vi "WPI_CANTalonSRX_Send.vi"(11 "Device ID (0)":u8) -> (3 "Device ID Out":u8)   [LabVIEW 2016]
uses:
  <vilib>/Rock Robotics/WPI/ThirdParty/CanMotor/TalonSRX/WPI_CANTalonSRX_GlobalOps.ctl
  <vilib>/Rock Robotics/WPI/ThirdParty/CanMotor/TalonSRX/WPI_CANTalonSRX_GlobalStatus.ctl
  <vilib>/Rock Robotics/WPI/ThirdParty/CanMotor/TalonSRX/WPI_CANTalonSRX_APIControlMode.ctl
  <vilib>/Rock Robotics/WPI/ThirdParty/CanMotor/TalonSRX/WPI_CANTalonSRX_ControlMode.ctl
  <vilib>/Rock Robotics/WPI/ThirdParty/CanMotor/TalonSRX/WPI_CANTalonSRX_MessageIDs.ctl
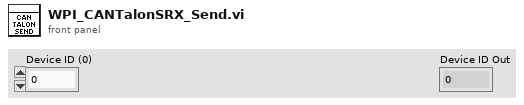
[diagram p1: front panel]
types:
  T1 = typedef "WPI_CANTalonSRX_APIControlMode.ctl" = enum8{"Percent VBus", "Speed", "Position", "Slave", "Unchanged / Invalid", "Voltage Compensation", "Current", "Motion Profile", "Motion Magic"}
  T2 = typedef "WPI_CANTalonSRX_GlobalOps.ctl" = enum16{"Read For Send", "Write After Receive General", "Write After Receive Feedback", "Write After Receive Encoder", "Write After Receive Ain", "Write Error", "Get All", "Set Output", "Set Mode", "Set Master ID", "Set Brake Mode", "Set Reverse Feedback Sensor", "Set Reverse Closed Loop Output", "Set Override Limits", "Set Forward Limit Enabled", "Set Reverse Limit Enabled", "Set Feedback Select", "Set Profile Select", "Set Throttle Ramp Rate", "Disable", "Set Enc Codes Per Rev", "Set Num Pot Turns", "Set Control Frame Rate", "Enable Legacy Control", "Write After Receive Pulse Width", "Set Enable Frame Rate", "Write After Receive Motion Profile", "Set Motion Profile Flow Control", "Set Motion Profile Control Frame Rate", "Set Current Limit Enable"}
  T3 = typedef "WPI_CANTalonSRX_GlobalStatus.ctl" = cluster{"Applied Throttle":dbl, "Module Enabled":bool, "CAN Error":errorcluster, "Closed Loop Error":dbl, "Forward Limit Switch Closed":bool, "Reverse Limit Switch Closed":bool, "Sensor Position":dbl, "Sensor Velocity":dbl, "Current":dbl, "Sticky Fault - Over Temp":bool, "Sticky Fault - Under Voltage":bool, "Sticky Fault - Forward Limit":bool, "Sticky Fault - Reverse Limit":bool, "Sticky Fault - Forward Soft Limit":bool, "Sticky Fault - Reverse Soft Limit":bool, "Brake is Enabled":bool, "Encoder Position":dbl, "Encoder Velocity":dbl, "Encoder Index Count":dbl, "Encoder A Pin State":bool, "Encoder B Pin State":bool, "Encoder Index Pin State":bool, "Analog In":dbl, "Analog In Velocity":dbl, "Temperature (C)":dbl, "Battery Voltage":dbl, "Control 5 Is Supported":bool, "Current Profile Slot Select":dbl, "Pos Div 8":bool, "Vel Div 4":bool, "Pulse Width Position":i32, "Pulse Width Velocity":i32, "Pulse Width Rise To Rise (us)":i32, "Pulse Width Rise To Fall (us)":i32, "Mot Prof Active Is Under Run":bool, "Mot Prof Active Has Under Run":bool, "Mot Prof Active Is Last":bool, "Mot Prof Active Velocity Only":bool, "Mot Prof Active Is Valid":bool, "Mot Prof Buffer Is Full":bool, "Mot Prof Active Profile Slot Select":i32, "Mot Prof NextID":i32, "Mot Prof Count":i32, "Mot Prof Active Velocity":dbl, "Mot Prof Active Position":dbl, "Mot Prof Output Enable":i32}
  T4 = typedef "WPI_CANTalonSRX_GlobalControl.ctl" = cluster{"Output":dbl, "Control Mode":T1, "Brake-Mode Override":T5, "Reverse Feedback Sensor":bool, "Reverse Closed-Loop Output":bool, "Override Limits":bool, "Forward Limit Enabled":bool, "Reverse Limit Enabled":bool, "Feedback Select":T6, "Profile Select":u8, "Master To Follow":u8, "Throttle Ramp Rate":u8, "Disabled":bool, "Encoder Codes Per Rev":u32, "Num Pot Turns":u32, "Control Frame Rate Ms":u8, "Use Control5 If Supported":bool, "Enable Frame Rate Ms":u8, "Motion Profile Flow Control":u8, "Motion Profile Control Frame Rate":u8, "Talon SRX Motion Profile Trajectory Point":T7, "Current Limit Enabled":bool}
  T5 = typedef "WPI_CANTalonSRX_BrakeOverride.ctl" = enum8{"No Override", "Override to Coast", "Override to Brake"}
  T6 = typedef "WPI_CANTalonSRX_FeedbackSelect.ctl" = u8
  T7 = typedef "WPI_CANTalonSRX_MotionProfileTrajectoryPt.ctl" = cluster{"Duration Ms":u8, "Velocity":dbl, "Position":dbl, "Profile Slot Select":u8, "Is Last":bool, "Velocity Only":bool, "Zero Position":bool, "Compress Code":u8, "Same Velocity":i32, "Delta Position":i32, "Count":u8}
  T8 = typedef "WPI_CANTalonSRX_ControlMode.ctl" = enum16{"Throttle (Duty-Cycle)", "Position Closed-Loop", "Velocity Closed-Loop", "Current Closed-Loop", "Voltage Compensation", "Slave Follower", "Motion Profile", "Motion Magic"}
  T9 = typedef "WPI_CANTalonSRX_MessageIDs.ctl" = u32
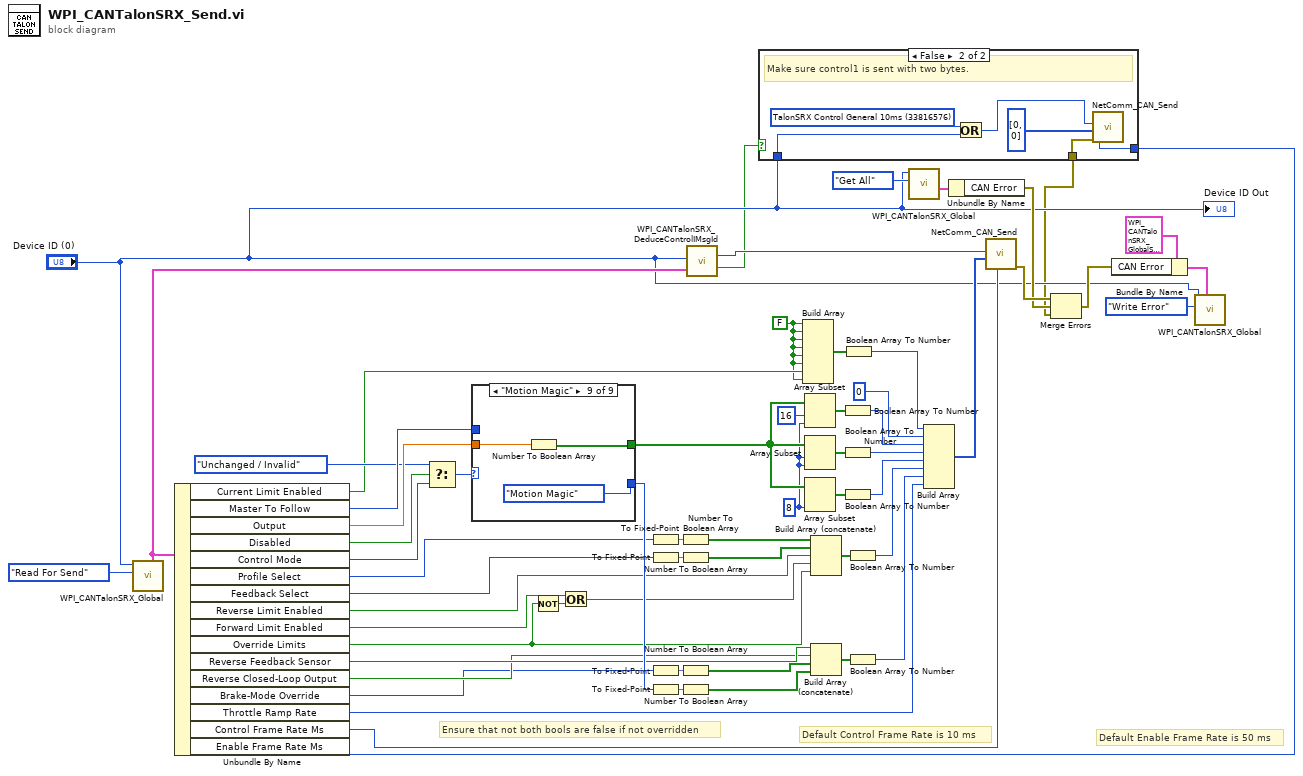
[diagram p0: block diagram]
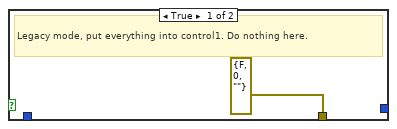
[diagram p2: hidden frame]
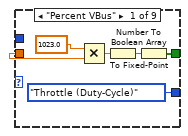
[diagram p3: hidden frame]
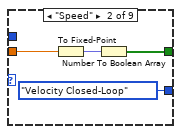
[diagram p4: hidden frame]
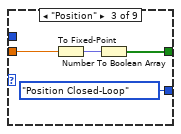
[diagram p5: hidden frame]
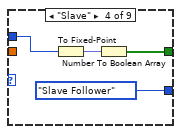
[diagram p6: hidden frame]
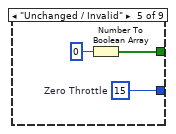
[diagram p7: hidden frame]
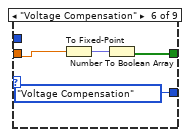
[diagram p8: hidden frame]
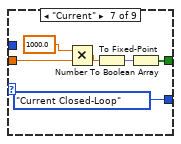
[diagram p9: hidden frame]
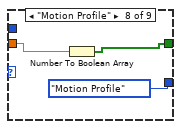
[diagram p10: hidden frame]
diagram:
  w3 = FALSE ("element")
  w44 = 8 ("length")
  # "Default Enable Frame Rate is 50 ms"
  # "Default Control Frame Rate is 10 ms"
  # "Ensure that not both bools are false if not overridden"
  n1 = call <vilib>:"WPI_CANTalonSRX_Global.vi"("Operation"=WPI_CANTalonSRX_GlobalOps."Read For Send", "Device ID (0)"="Device ID (0)") -> ("Read For Send"=w11:T4)  [unwired: 7 in, 2 out]
  n2 = Unbundle By Name(w11) -> ("Current Limit Enabled"=w4:bool, "Master To Follow"=w23:u8, "Output"=w59:dbl, "Disabled"=w15:bool, "Control Mode"=w25:T1, "Profile Select"=w30:u8, "Feedback Select"=w29:T6, "Reverse Limit Enabled"=w33:bool, "Forward Limit Enabled"=w34:bool, "Override Limits"=w31:bool, "Reverse Feedback Sensor"=w28:bool, "Reverse Closed-Loop Output"=w27:bool, "Brake-Mode Override"=w26:T5, "Throttle Ramp Rate"=w22:u8, "Control Frame Rate Ms"=w13:u8, "Enable Frame Rate Ms"=w7:u8)
  n3 = Select(t=WPI_CANTalonSRX_APIControlMode."Unchanged / Invalid", s=w15, f=w25) -> (s? t:f=w16:T1)
  n4 = case shown="\"Motion Magic\"" w16 {
    tunnel: w59 -> [w67 w71 w75 _ _ w83 w89 w93 w97]
    tunnel: [WPI_CANTalonSRX_ControlMode."Throttle (Duty-Cycle)" WPI_CANTalonSRX_ControlMode."Velocity Closed-Loop" WPI_CANTalonSRX_ControlMode."Position Closed-Loop" WPI_CANTalonSRX_ControlMode."Slave Follower" w80 WPI_CANTalonSRX_ControlMode."Voltage Compensation" WPI_CANTalonSRX_ControlMode."Current Closed-Loop" WPI_CANTalonSRX_ControlMode."Motion Profile" WPI_CANTalonSRX_ControlMode."Motion Magic" ("Talon SRX Mode")] -> w50
    tunnel: [w65 w69 w73 w78 w82 w84 w91 w95 w96] -> w45
    tunnel: w23 -> [_ _ _ w76 _ _ _ _ _]
    frame "Percent VBus" {
      n5 = Multiply(x=1023.0 ("y"), y=w67) -> (x*y=w63:dbl)
      n6 = To Fixed-Point(number=w63) -> (fixed-point=w62:fxp<+/-,24,24>)  [unwired: 1 in]
      n7 = Number To Boolean Array(number=w62) -> (Boolean array=w65:bool[])
    }
    frame "Speed" {
      n8 = To Fixed-Point(number=w71) -> (fixed-point=w68:fxp<+/-,24,24>)  [unwired: 1 in]
      n9 = Number To Boolean Array(number=w68) -> (Boolean array=w69:bool[])
    }
    frame "Position" {
      n10 = To Fixed-Point(number=w75) -> (fixed-point=w72:fxp<+/-,24,24>)  [unwired: 1 in]
      n11 = Number To Boolean Array(number=w72) -> (Boolean array=w73:bool[])
    }
    frame "Slave" {
      n12 = To Fixed-Point(number=w76) -> (fixed-point=w77:fxp<+,6,6>)  [unwired: 1 in]
      n13 = Number To Boolean Array(number=w77) -> (Boolean array=w78:bool[])
    }
    frame "Unchanged / Invalid" {
      w80 = 15  # Zero Throttle
      n14 = Number To Boolean Array(number=0 ("index")) -> (Boolean array=w82:bool[])
    }
    frame "Voltage Compensation" {
      n15 = To Fixed-Point(number=w83) -> (fixed-point=w85:fxp<+/-,24,16>)  [unwired: 1 in]
      n16 = Number To Boolean Array(number=w85) -> (Boolean array=w84:bool[])
    }
    frame "Current" {
      n17 = Multiply(x=1000.0, y=w89) -> (x*y=w87:dbl)
      n18 = To Fixed-Point(number=w87) -> (fixed-point=w92:fxp<+/-,24,24>)  [unwired: 1 in]
      n19 = Number To Boolean Array(number=w92) -> (Boolean array=w91:bool[])
    }
    frame "Motion Profile" {
      n20 = Number To Boolean Array(number=w93) -> (Boolean array=w95:bool[])
    }
    frame "Motion Magic" {
      n21 = Number To Boolean Array(number=w97) -> (Boolean array=w96:bool[])
    }
  }
  n22 = Not(x=w31) -> (.not. x?=w24:bool)
  n23 = Or(x=w34, y=w24) -> (x .or. y?=w32:bool)
  n24 = To Fixed-Point(number=w30) -> (fixed-point=w6:fxp<+,1,1>)  [unwired: 1 in]
  n25 = To Fixed-Point(number=w29) -> (fixed-point=w42:fxp<+,4,4>)  [unwired: 1 in]
  n26 = To Fixed-Point(number=w26) -> (fixed-point=w38:fxp<+,2,2>)  [unwired: 1 in]
  n27 = To Fixed-Point(number=w50) -> (fixed-point=w51:fxp<+,4,4>)  [unwired: 1 in]
  n28 = Number To Boolean Array(number=w6) -> (Boolean array=w35:bool[])
  n29 = Number To Boolean Array(number=w42) -> (Boolean array=w41:bool[])
  n30 = Number To Boolean Array(number=w38) -> (Boolean array=w37:bool[])
  n31 = Number To Boolean Array(number=w51) -> (Boolean array=w36:bool[])
  n32 = call <vilib>:"WPI_CANTalonSRX_DeduceControlIMsgId.vi"("Device ID (0)"="Device ID (0)", "Read For Send"=w11) -> ("Control ArbID"=w12:u32, "Using Legacy Frame"=w9:bool)  [unwired: 12 in]
  n33 = case shown="False" w9 {
    tunnel: "Device ID (0)" -> [_ w103]
    tunnel: [errorcluster {"status"=FALSE, "code"=0, "source"=""} ("error out") w102] -> w8
    tunnel: w7 -> [_ w100]
    frame True {
      # "Legacy mode, put everything into control1. Do nothing here."
    }
    frame False {
      w104 = T9 33816576 items=["TalonSRX Control General 10ms"=33816576, "TalonSRX Control Rates Slow"=33816640, "TalonSRX Control ClearFlags Slow"=33816704, "TalonSRX Status General 10ms"=33821696, "TalonSRX Status Feedback 20ms"=33821760, "TalonSRX Status Enc 100ms"=33821824, "TalonSRX Status AinTempVbat 100ms"=33821888, "TalonSRX Status Startup Once"=33821952, "TalonSRX Status Debug"=33822080, "TalonSRX Config SetGainsSlot0 A"=33823808, "TalonSRX Config SetGainsSlot0 B"=33823872, "TalonSRX Config SetGainsSlot1 A"=33823936, "TalonSRX Config SetGainsSlot1 B"=33824000, "TalonSRX Config SetSoftLimits"=33824064, "TalonSRX Config WebControl"=33824128, "TalonSRX Param Request"=33822720, "TalonSRX Param Response"=33822784, "TalonSRX Param Set"=33822848]
      # "Make sure control1 is sent with two bytes."
      n34 = Or(x=w104, y=w103) -> (x .or. y?=w105:T9)
      n35 = call <vilib>:"NetComm_CAN_Send.vi"("Period (ms)"=w100, "Data"=u8[] [0, 0] ("Token Space"), "Message ID"=w105) -> ("error out"=w102:errorcluster)  [unwired: 8 in]
    }
  }
  n36 = Build Array(w3, w3, w3, w3, w3, w3, w4, w3) -> (w2:bool[])
  n37 = Array Subset(array=w45, index=16, length=w44) -> (w46:bool[])
  n38 = Array Subset(array=w45, index=w44, length=w44) -> (w48:bool[])
  n39 = Array Subset(array=w45, length=w44) -> (w47:bool[])  [unwired: 1 in]
  n40 = Build Array (concatenate)(w35, w41, w33, w32, w31) -> (w40:bool[])
  n41 = Build Array (concatenate)(w28, w27, w37, w36) -> (w52:bool[])
  n42 = Boolean Array To Number(Boolean array=w46) -> (number=w49:u32)
  n43 = Boolean Array To Number(Boolean array=w48) -> (number=w54:u32)
  n44 = Boolean Array To Number(Boolean array=w47) -> (number=w53:u32)
  n45 = Boolean Array To Number(Boolean array=w2) -> (number=w1:u8)
  n46 = Boolean Array To Number(Boolean array=w40) -> (number=w39:u32)
  n47 = Boolean Array To Number(Boolean array=w52) -> (number=w55:u32)
  n48 = call <vilib>:"WPI_CANTalonSRX_Global.vi"("Operation"=WPI_CANTalonSRX_GlobalOps."Get All", "Device ID (0)"="Device ID (0)") -> ("Get All"=w18:T3)  [unwired: 7 in, 2 out]
  n49 = Build Array(w1, u8 0, w49, w54, w53, w39, w55, w22) -> (w61:u32[])
  n50 = Unbundle By Name(w18) -> ("CAN Error"=w17:errorcluster)
  n51 = call <vilib>:"NetComm_CAN_Send.vi"("Period (ms)"=w13, "Data"=w61, "Message ID"=w12) -> ("error out"=w21:errorcluster)  [unwired: 8 in]
  n52 = Merge Errors(w21, w17, w8) -> (w20:errorcluster)
  n53 = Bundle By Name(cluster=T3 {"Applied Throttle"=0.0, "Module Enabled"=FALSE, "CAN Error"={"status"=FALSE, "code"=0, "source"=""}, "Closed Loop Error"=0.0, "Forward Limit Switch Closed"=FALSE, "Reverse Limit Switch Closed"=FALSE, "Sensor Position"=0.0, "Sensor Velocity"=0.0, "Current"=0.0, "Sticky Fault - Over Temp"=FALSE, "Sticky Fault - Under Voltage"=FALSE, "Sticky Fault - Forward Limit"=FALSE, "Sticky Fault - Reverse Limit"=FALSE, "Sticky Fault - Forward Soft Limit"=FALSE, "Sticky Fault - Reverse Soft Limit"=FALSE, "Brake is Enabled"=FALSE, "Encoder Position"=0.0, "Encoder Velocity"=0.0, "Encoder Index Count"=0.0, "Encoder A Pin State"=FALSE, "Encoder B Pin State"=FALSE, "Encoder Index Pin State"=FALSE, "Analog In"=0.0, "Analog In Velocity"=0.0, "Temperature (C)"=0.0, "Battery Voltage"=0.0, "Control 5 Is Supported"=FALSE, "Current Profile Slot Select"=0.0, "Pos Div 8"=FALSE, "Vel Div 4"=FALSE, "Pulse Width Position"=0, "Pulse Width Velocity"=0, "Pulse Width Rise To Rise (us)"=0, "Pulse Width Rise To Fall (us)"=0, "Mot Prof Active Is Under Run"=FALSE, "Mot Prof Active Has Under Run"=FALSE, "Mot Prof Active Is Last"=FALSE, "Mot Prof Active Velocity Only"=FALSE, "Mot Prof Active Is Valid"=FALSE, "Mot Prof Buffer Is Full"=FALSE, "Mot Prof Active Profile Slot Select"=0, "Mot Prof NextID"=0, "Mot Prof Count"=0, "Mot Prof Active Velocity"=0.0, "Mot Prof Active Position"=0.0, "Mot Prof Output Enable"=0} ("Write After Receive"), "CAN Error"=w20) -> (w56:T3)
  n54 = call <vilib>:"WPI_CANTalonSRX_Global.vi"("Write After Receive"=w56, "Operation"=WPI_CANTalonSRX_GlobalOps."Write Error", "Device ID (0)"="Device ID (0)") -> ()  [unwired: 6 in, 3 out]
  "Device ID Out" <- "Device ID (0)"
